vi "Arrow_Set.vi"   [LabVIEW 2020]
uses:
  Globals/Arrow_Globals.vi
  Arrow_Control_States.ctl
types:
  T1 = typedef "Arrow_Control_States.ctl" = enum16{"No-Op", "GoToAngle", "Manual_%Vbus"}
  T2 = typedef "Arrow_Cluster.ctl" = cluster{"Control_States":T1, "Manual_Throttle":dbl, "Angle_Goal":dbl}
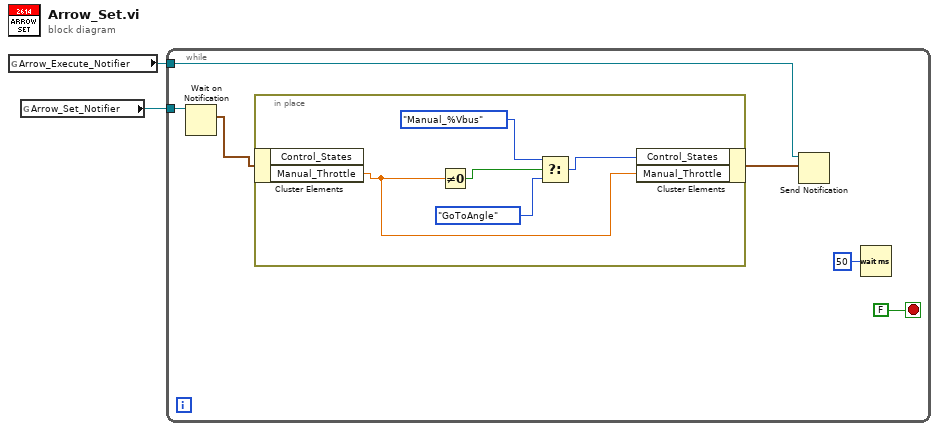
[diagram p0: block diagram]
diagram:
  n1 = global read "Arrow_Globals.vi" "Arrow_Execute_Notifier"() -> (w1:refnum<notifier>)
  n2 = global read "Arrow_Globals.vi" "Arrow_Set_Notifier"() -> (w2:refnum<notifier>)
  n3 = while {
    tunnel: w2 -> [w8]
    tunnel: w1 -> [w5]
    stop <- FALSE stop-if-true
    n4 = Wait on Notification(notifier=w8) -> (notification=w4:T2)  [unwired: 3 in, 3 out]
    n5 = in-place {
      n6 = in-place-cluster #1(w4) -> ("Manual_Throttle"=w9:dbl)  [unwired: 1 out]
      n7 = Not Equal To 0?(x=w9) -> (x != 0?=w13:bool)
      n8 = Select(t=Arrow_Control_States."Manual_%Vbus" ("Control_States"), s=w13, f=Arrow_Control_States."GoToAngle" ("Control_States")) -> (s? t:f=w10:T1)
      n9 = in-place-cluster #1("Control_States"=w10, "Manual_Throttle"=w9) -> (w3:T2)
    }
    n10 = Send Notification(notification=w3, notifier=w5) -> ()  [unwired: 1 in, 2 out]
    n11 = Wait (ms)(milliseconds to wait=u32 50) -> ()  [unwired: 1 out]
  }
